vi "MUX Initialization SubVI.vi"(4 "Topology Name":string, 5 "Channels Array":string[](array[string]), 6 "Resource Name":string, 7 "Decimation":i32, 8 "error in (no error)":errorcluster, 9 "Custom XML":string, 11 "Device Item Ref in":T1 format="%.0x") -> (0 "error out":errorcluster, 3 "Device Item Ref out":T1 format="%.0x")   [LabVIEW 2013, in "MUX Custom Device.lvlib"]
uses:
  MUX Custom Device.lvlib
  <vilib>/NI Veristand/Custom Device API/Custom Device Item Ref.ctl
  <vilib>/NI Veristand/Custom Device API/Custom Device Channel.ctl
  <vilib>/NI Veristand/Custom Device API/Custom Device Channel Type.ctl
  MUX Global.vi
  <vilib>/NI Veristand/Custom Device API/Set Item Property (String).vi
  <vilib>/NI Veristand/Custom Device API/Custom Device API.lvlib
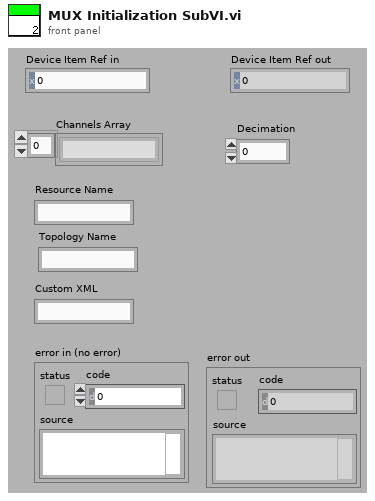
[diagram p1: front panel]
types:
  T1 = typedef "Custom Device API.lvlib/Custom Device Item Ref.ctl" = u64
  T2 = typedef "Custom Device API.lvlib/Custom Device Channel.ctl" = cluster{"Type":T3, "Units":string, "Default Value":dbl, "Faultable":bool, "Scalable":bool}
  T3 = typedef "Custom Device API.lvlib/Custom Device Channel Type.ctl" = enum16{"Input", "Output"}
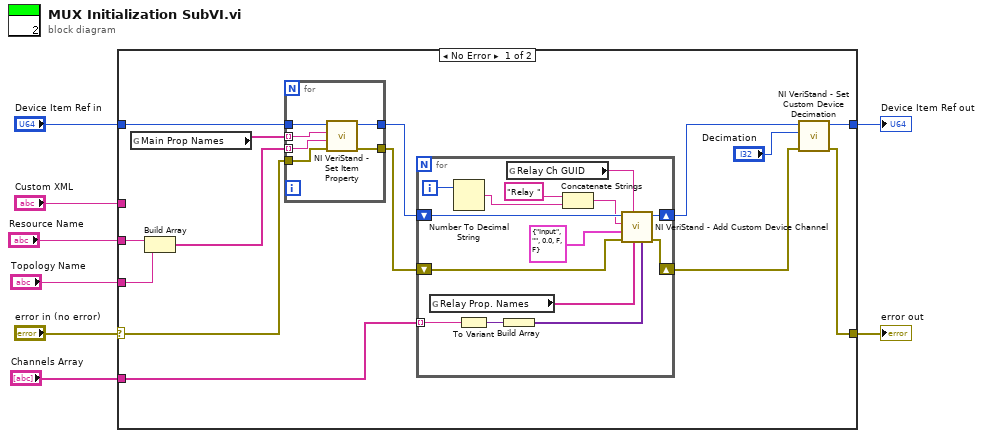
[diagram p0: block diagram]
diagram:
  n1 = case shown="No Error" "error in (no error)" {
    selector: "error in (no error)" -> [w12 w44]
    tunnel: [w18 w44] -> w4
    tunnel: [w21 w43] -> w6
    tunnel: "Device Item Ref in" -> [w17 w43]
    tunnel: "Custom XML" -> [_ _]
    tunnel: "Channels Array" -> [w22 _]
    tunnel: "Resource Name" -> [w15 _]
    tunnel: "Topology Name" -> [w14 _]
    frame No Error {
      n2 = global read "MUX Global.vi" "Main Prop Names"() -> (w16:string[])
      n3 = Build Array(w15, w14) -> (w13:string[])
      n4 = for {
        tunnel: w17 -> [w28]
        tunnel: [w27] -> w10
        tunnel: w16 -> [w26] mode=indexing
        tunnel: w13 -> [w25] mode=indexing
        tunnel: w12 -> [w24]
        tunnel: [w23] -> w11
        n5 = call-poly <vilib>:"NI VeriStand - Set Item Property.vi"("error in (no error)"=w24, "Value"=w25, "Property Name"=w26, "Item Ref in"=w28) -> ("error out"=w23:errorcluster, "Item Ref out"=w27:T1)  [unwired: 5 in, 1 out]
      }
      n6 = for {
        tunnel: w22 -> [w41] mode=indexing
        shift-right: [w35] -> w19
        shift-left: w11 -> [w36]
        shift-right: [w30] -> w9
        shift-left: w10 -> [w42]
        i -> [w29]
        n7 = global read "MUX Global.vi" "Relay Prop. Names"() -> (w32:string[])
        n8 = Number To Decimal String(number=w29) -> (decimal integer string=w39:string)  [unwired: 1 in]
        n9 = To Variant(anything=w41) -> (Variant=w34:variant)
        n10 = Build Array(w34) -> (w33:variant[])
        n11 = global read "MUX Global.vi" "Relay Ch GUID"() -> (w37:string)
        n12 = Concatenate Strings("Relay ", w39) -> (w38:string)
        n13 = call <vilib>:"NI VeriStand - Add Custom Device Channel.vi"("Property Values"=w33, "Property names"=w32, "GUID (Default Channel)"=w37, "error in (no error)"=w36, "Channel"=T2 {"Type"=enum."Input", "Units"="", "Default Value"=0.0, "Faultable"=FALSE, "Scalable"=FALSE}, "Channel Name"=w38, "Parent Ref in"=w42) -> ("error out"=w35:errorcluster, "Parent Ref out"=w30:T1)  [unwired: 1 in, 2 out]
      }
      n14 = call <vilib>:"NI VeriStand - Set Custom Device Decimation.vi"("error in (no error)"=w19, "Decimation"="Decimation", "Device Ref in"=w9) -> ("error out"=w18:errorcluster, "Device Ref out"=w21:T1)  [unwired: 7 in]
    }
    frame Error {
    }
  }
  "error out" <- w4
  "Device Item Ref out" <- w6
